vi "Ex1v2.vi"() -> ()   [LabVIEW 2017]
panel:
  out "LED 5":bool
  out "LED 4":bool
  out "LED 3":bool
  out "LED2":bool
  out "LED1":bool
  in  "Délai":dbl(knob) scale=1.0..1000.0
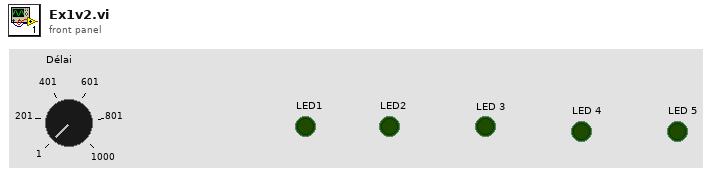
[diagram p1: front panel]
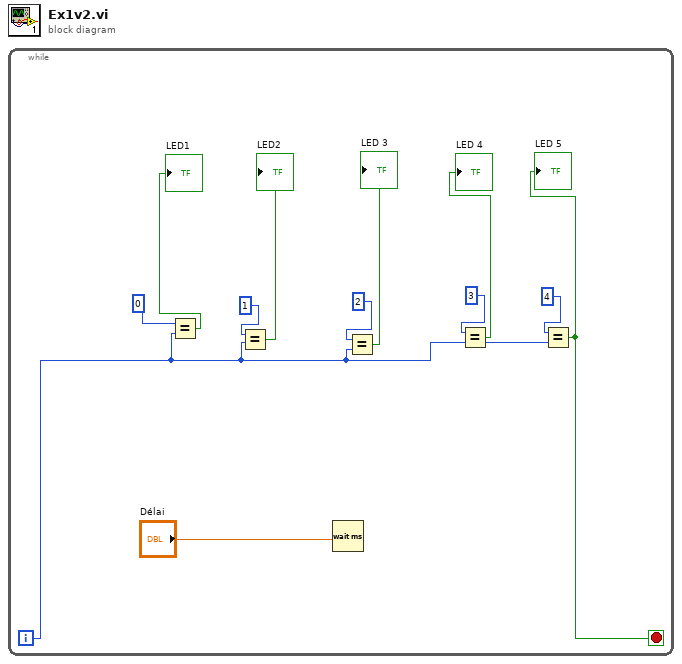
[diagram p0: block diagram]
diagram:
  n1 = while {
    i -> [w2]
    stop <- w1 stop-if-true
    n2 = Equal?(x=0, y=w2) -> (x = y?=→"LED1":bool)
    n3 = Equal?(x=1, y=w2) -> (x = y?=→"LED2":bool)
    n4 = Wait (ms)(milliseconds to wait="Délai") -> ()  [unwired: 1 out]
    n5 = Equal?(x=2, y=w2) -> (x = y?=→"LED 3":bool)
    n6 = Equal?(x=3, y=w2) -> (x = y?=→"LED 4":bool)
    n7 = Equal?(x=4, y=w2) -> (x = y?=w1:bool)
    "LED 5" <- w1
  }
